vi "SampleVI.vi"() -> ()   [LabVIEW 2019, in "LabJSON.lvlib"]
uses:
  LabJSON.lvlib
panel:
  out "Sum":dbl
  in  "Checkbox":bool
  in  "File Path Control":path
  in  "Numeric":dbl
  in  "Array - String":string[][](array[string])
  in  "Cluster":T1={"Numeric"=1.0, "String"="One", "Checkbox"=FALSE}
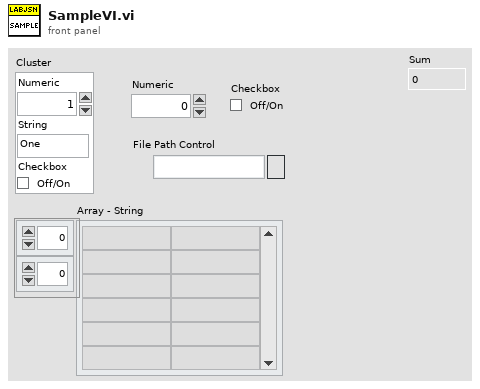
[diagram p1: front panel]
types:
  T1 = cluster{"Numeric":dbl, "String":string, "Checkbox":bool}
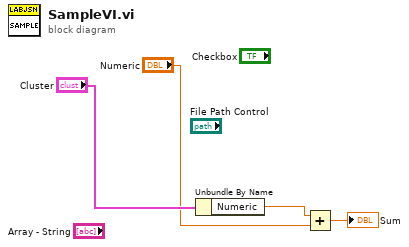
[diagram p0: block diagram]
diagram:
  n1 = Unbundle By Name("Cluster") -> ("Numeric"=w3:dbl)
  n2 = Add(x=w3, y="Numeric") -> (x+y=→"Sum":dbl)
